vi "Orca Flash Data Spooler.vi"(7 "Calling VI Ref":refnum<vi>) -> ()   [LabVIEW 2016]
uses:
  <vilib>/vision/Image Controls.llb/IMAQ Image.ctl
  Orca Flash Capture Manager Controls/Orca Flash Capture Notifier Type.ctl
  Orca Flash Capture Manager Controls/Orca Flash Capture Actions.ctl
  Orca Flash Capture Manager Controls/Orca Flash Capture Switch Line Scan Modes.ctl
  Orca Flash Data Spooler/Orca Data Spooler Type Defs/Orca Data Spooler Notifier Type.ctl
  Orca Flash Data Spooler/Orca Data Spooler Type Defs/Orca Data Spooler Actions.ctl
  <vilib>/Utility/miscctls.llb/LVPointTypeDef.ctl
  Orca Flash Data Spooler/Orca Data Spooler Type Defs/Orca Data Spooler Last Used.ctl
  Tools/Copy File with Progress/Copy File DLL/x64/Debug/Copy File DLL.dll
panel:
  out "Transfer Amount (%)":u8
  out "Current File":string
  out "Copy Success":bool
  in  "Abort":bool
  in  "Skip File":bool
  in  "Auto Match Paths":bool=TRUE
  in  "Disable Spooler":bool
  in  "Set Destination":bool
  in  "Quit":bool
  out "Destination Path":string
  out "Source Path":string
  out "Start Up Error":errorcluster
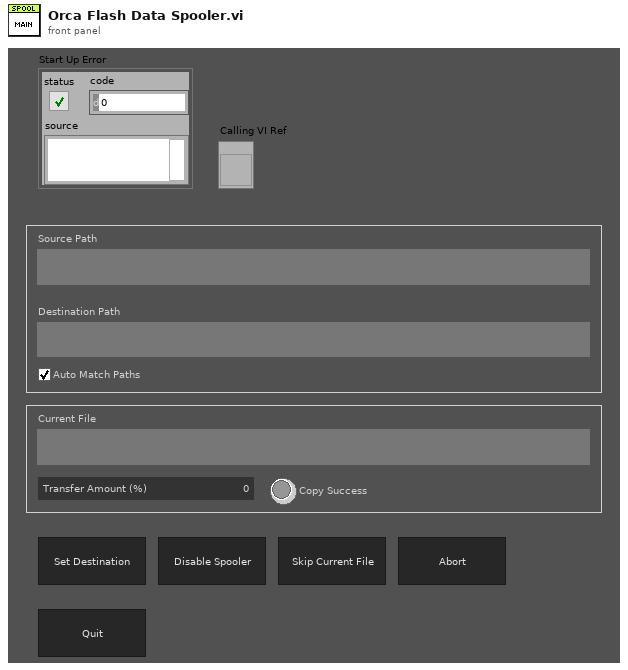
[diagram p1: front panel]
types:
  T1 = enum16{"Always On", "Always Off", "Off While Running"}
  T2 = typedef "LVPointTypeDef.ctl" = cluster{"Horizontal":i16, "Vertical":i16}
  T3 = typedef "Orca Data Spooler Actions.ctl" = enum16{"Idle", "Start Spooler", "Update Destination", "Wait for File", "Copy File", "Copy JSON Files", "Abort", "Exit", "Quit"}
  T4 = typedef "Orca Data Spooler Notifier Type.ctl" = cluster{"Actions":T3, "Source":path, "Destination":path, "Running?":bool}
  T5 = enum8{"Enabled", "Disabled", "Disabled and Grayed Out"}
  T6 = typedef "Orca Flash Capture Notifier Type.ctl" = cluster{"Actions":T7, "Running?":bool, "Preview Exposure (s)":dbl, "Capture Exposure (s)":dbl, "Cycles":u16, "Frames":u32, "No. of Z Steps":u16, "Z Step Size (µm)":dbl, "Base Path":path, "Init Z Position (µm)":dbl, "Lasers Lines":string[], "Save Path":path, "Line Scan?":bool, "Line Scan Mode":T8, "Collect Metadata?":bool}
  T7 = typedef "Orca Flash Capture Actions.ctl" = enum16{"Idle", "Live Preview", "Capture", "Laser On", "Laser Off", "Open Shutters", "Close Shutters", "Set Exposure Time", "Start Acquisition", "Update SubFolder", "Write Metadata", "Setup", "Camera", "Switch", "Step", "Cycle", "External Cycle Sync", "Abort", "Quit"}
  T8 = typedef "Orca Flash Capture Switch Line Scan Modes.ctl" = enum32{"Automatic", "Use Presets", "Manual"}
  T9 = typedef "IMAQ Image.ctl" = refnum<image>
  T10 = cluster{"Image Ref":T9, "Cycle Number":u16, "Camera Running?":bool, "Capture?":bool}
  T11 = enum32{"Bad", "Idle", "Run top level", "Running"}
  T12 = typedef "Orca Data Spooler Last Used.ctl" = cluster{"Source":string, "Destination":string}
  T13 = typedef "LVRectTypeDef.ctl" = cluster{"Left":i16, "Top":i16, "Right":i16, "Bottom":i16}
  T14 = typedef "LVBoundsTypeDef.ctl" = cluster{"Width":u32, "Height":u32}
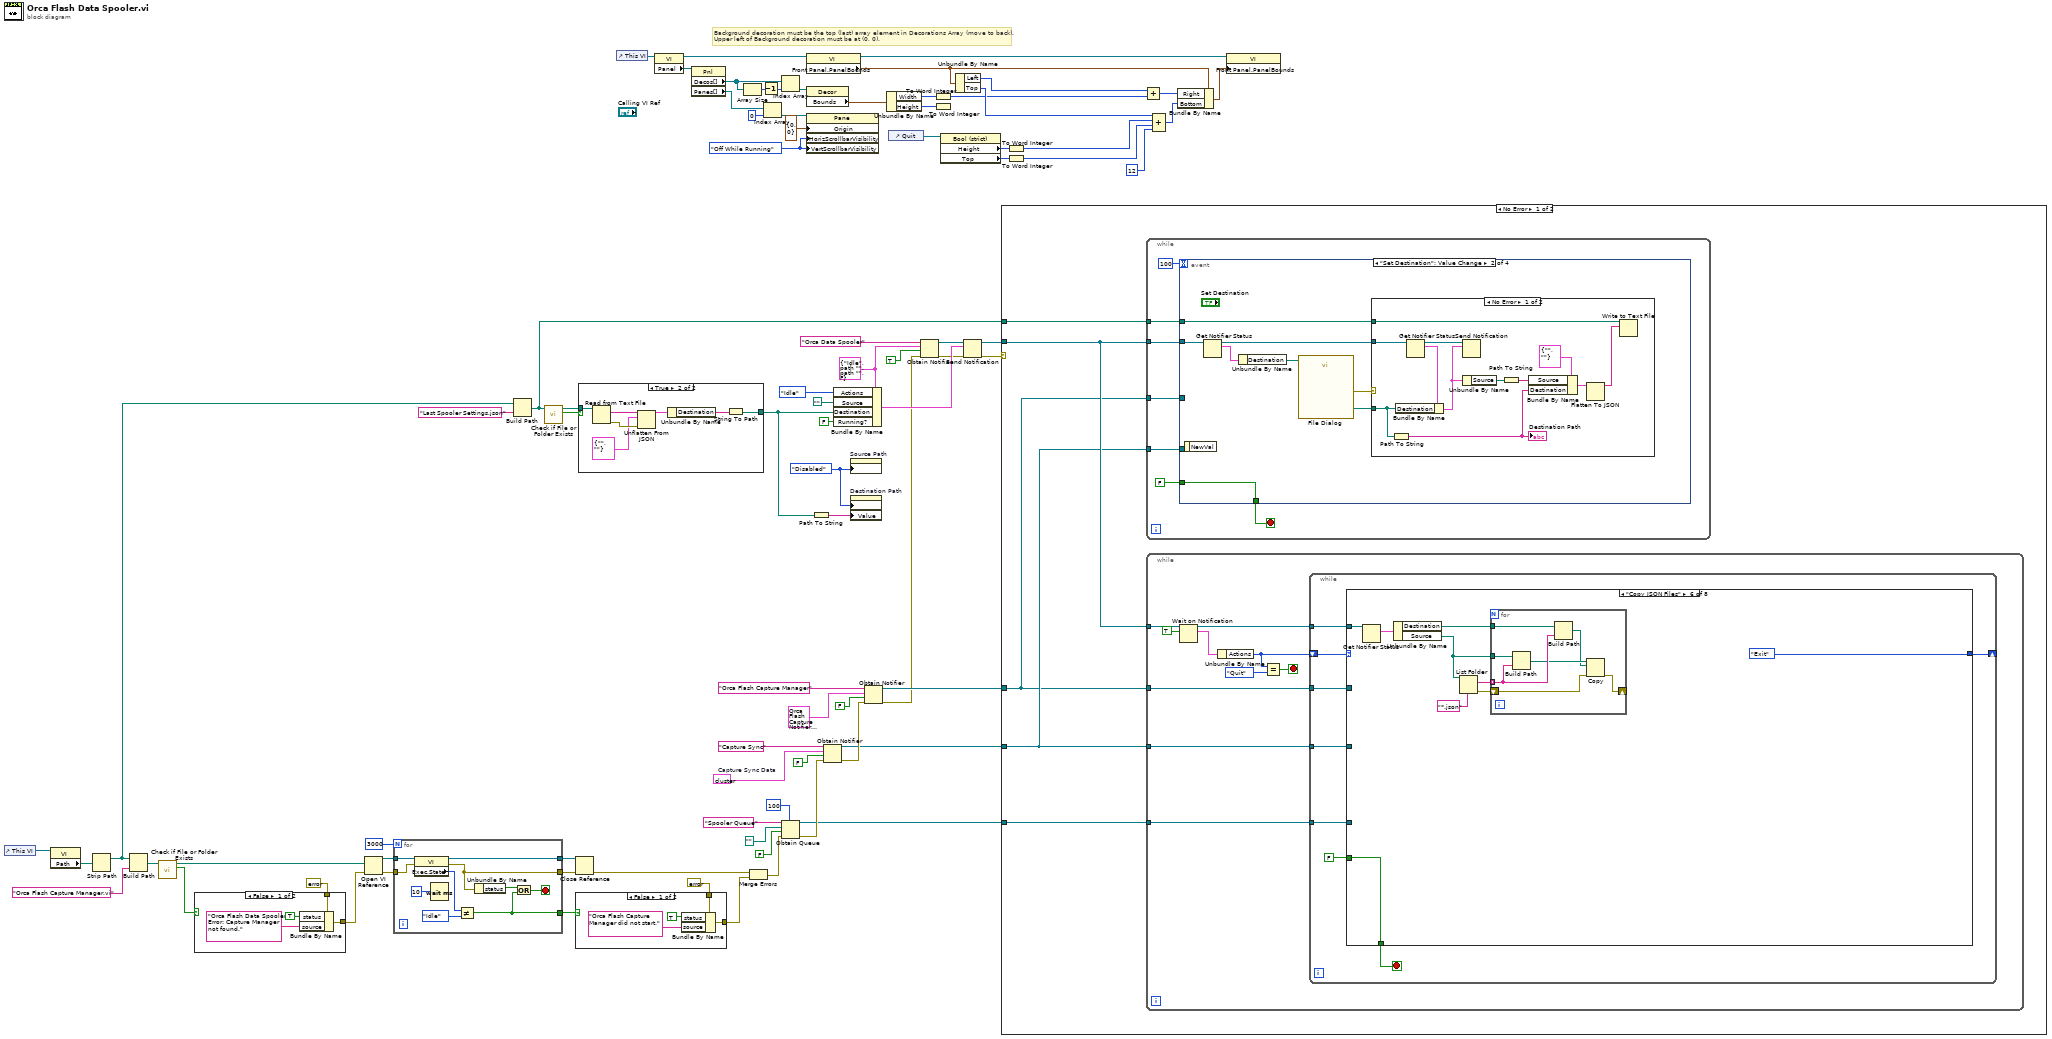
[diagram p0: block diagram]
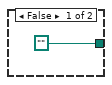
[diagram p2: hidden frame]
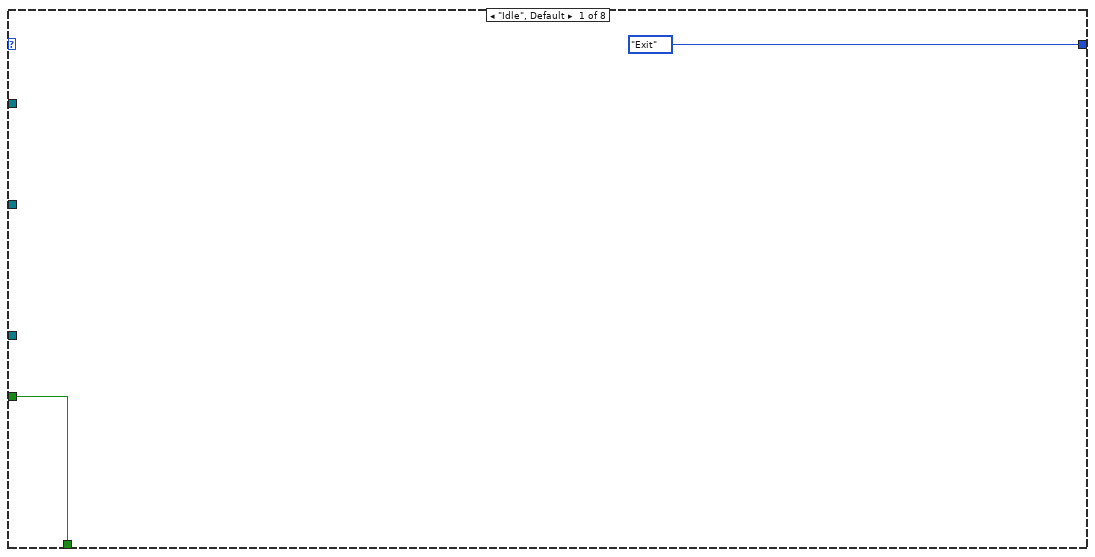
[diagram p3: hidden frame]
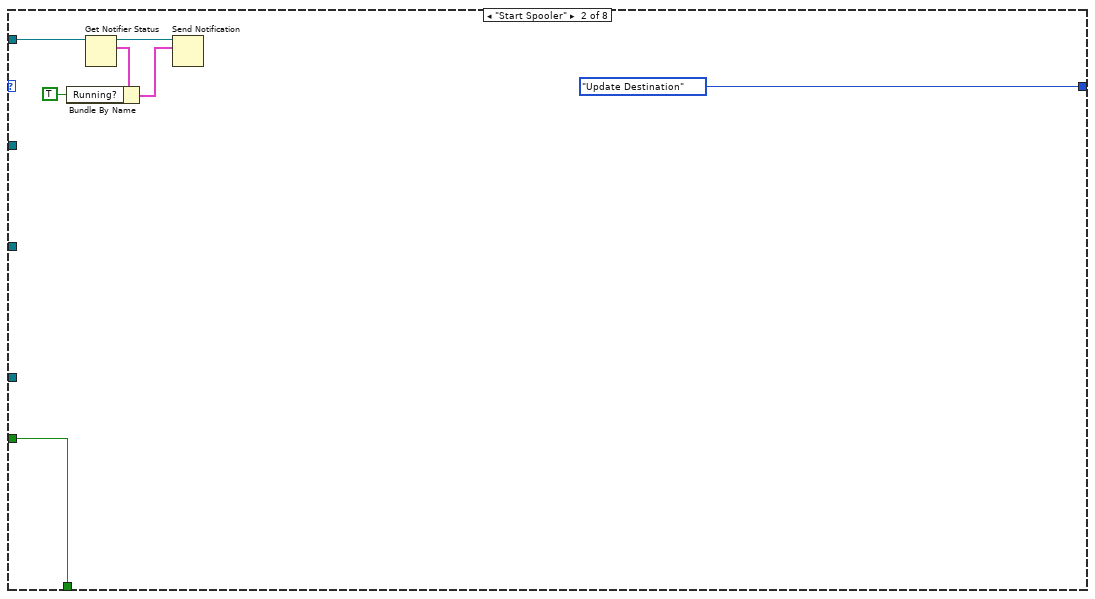
[diagram p4: hidden frame]
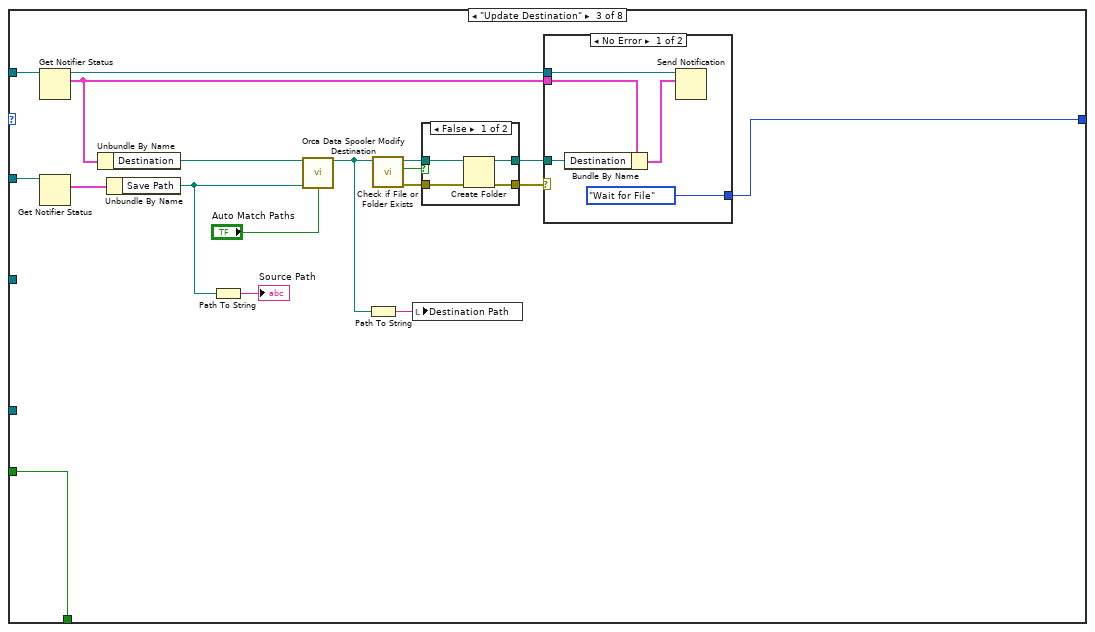
[diagram p5: hidden frame]
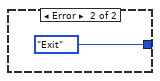
[diagram p6: hidden frame]
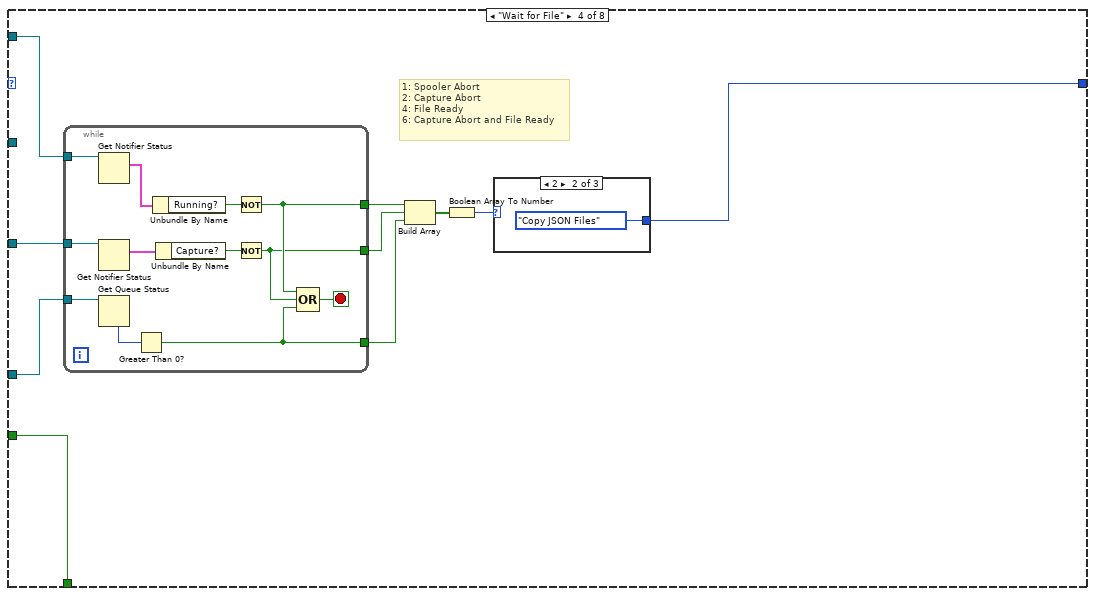
[diagram p8: hidden frame]
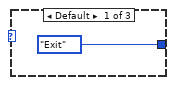
[diagram p9: hidden frame]
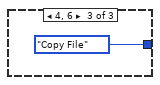
[diagram p10: hidden frame]
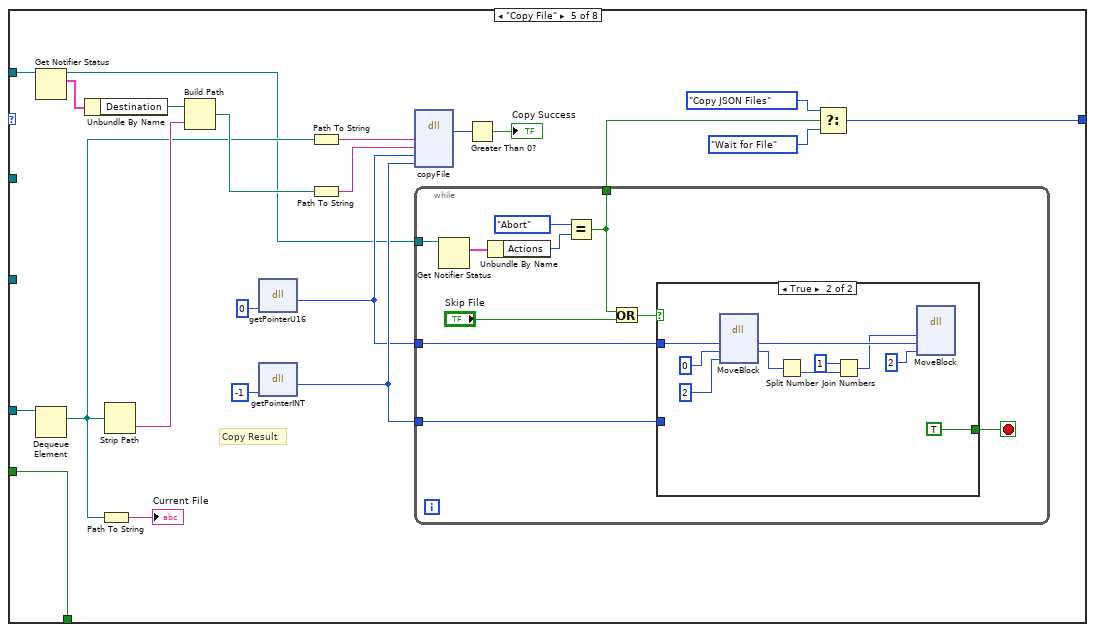
[diagram p11: hidden frame]
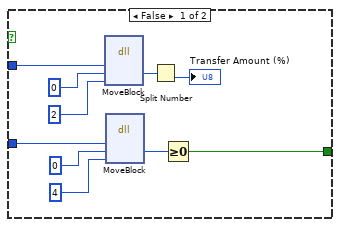
[diagram p12: hidden frame]
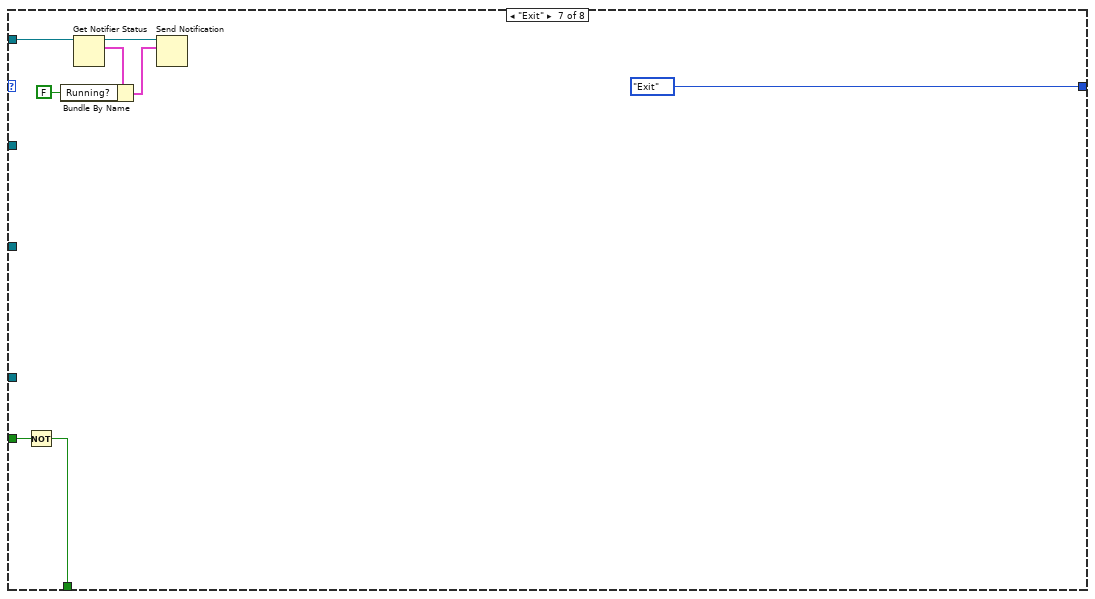
[diagram p13: hidden frame]
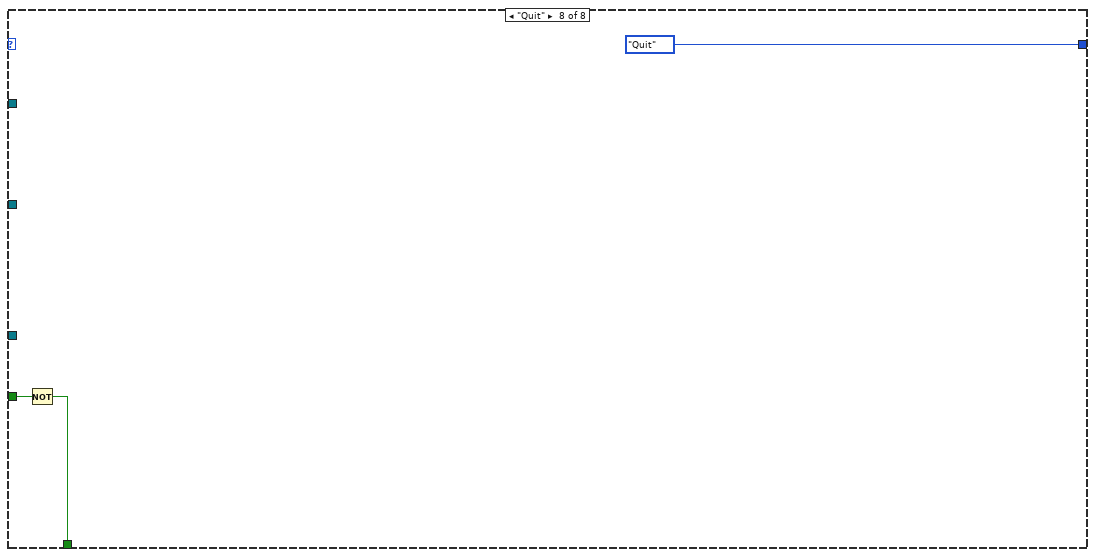
[diagram p14: hidden frame]
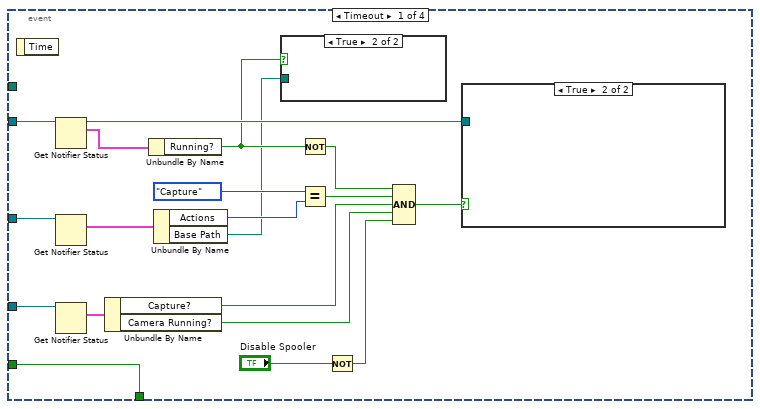
[diagram p15: hidden frame]
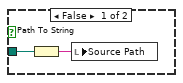
[diagram p16: hidden frame]
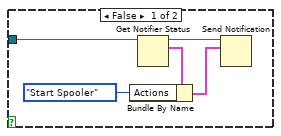
[diagram p17: hidden frame]
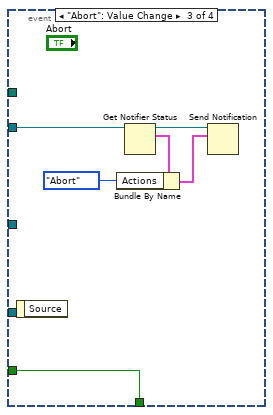
[diagram p19: hidden frame]
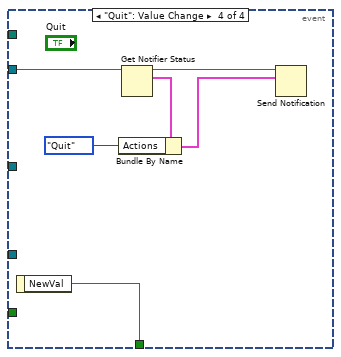
[diagram p20: hidden frame]
diagram:
  w21 = T1."Off While Running" ("Vertical Scrollbar Visibility")
  w47 = T4 {"Actions"=enum."Idle", "Source"=path "", "Destination"=path "", "Running?"=FALSE} ("Orca Data Spooler Notifier Type")
  w54 = T5."Disabled" ("Disabled")
  w69 = T10 {"Image Ref"=refnum, "Cycle Number"=0, "Camera Running?"=FALSE, "Capture?"=FALSE}  # Capture Sync Data
  # "Background decoration must be the top (last) array element in Decorations Array (move to back).\nUpper left of Background decoration must be at (0, 0)."
  n1 = control-ref of="This VI"() -> (w82:refnum<vi>)
  n2 = property class="VI"(reference=w82) -> ("Path"=w81:path)  [unwired: 1 in, 2 out]
  n3 = Strip Path(path=w81) -> (stripped path=w52:path)  [unwired: 1 out]
  n4 = Build Path(base path=w52, name or relative path="Orca Flash Capture Manager.vi" ("name (unnamed)")) -> (appended path=w79:path)
  n5 = call <vilib>:"Check if File or Folder Exists.vi"("path"=w79) -> ("file or folder exists?"=w78:bool, "dup path"=w75:path)  [unwired: 8 in, 1 out]
  n6 = case shown="False" w78 {
    tunnel: errorcluster {"status"=FALSE, "code"=0, "source"=""} ("error in (no error)") -> [w84 w87]
    tunnel: [w83 w87] -> w74
    frame False {
      n7 = Bundle By Name(cluster=w84, "status"=TRUE, "source"="Orca Flash Data Spooler Error: Capture Manager not found." ("name (unnamed)")) -> (w83:errorcluster)
    }
    frame True {
    }
  }
  n8 = Open VI Reference(vi path=w75, error in (no error)=w74) -> (vi reference=w76:refnum<vi>, error out=w70:errorcluster)  [unwired: 4 in]
  n9 = for {
    N: 3000 -> [_]
    tunnel: w76 -> [w97]
    tunnel: [w93] -> w72
    tunnel: [w88] -> w62
    tunnel: [w90] -> w71
    tunnel: w70 -> [w89]
    stop <- w91 stop-if-true
    n10 = property class="VI"(reference=w97, error in=w89) -> (reference out=w93:refnum<vi>, error out=w90:errorcluster, "Exec.State"=w95:T11)
    n11 = Wait (ms)(milliseconds to wait=u32 10) -> ()  [unwired: 1 out]
    n12 = Not Equal?(x=w95, y=T11."Idle") -> (x != y?=w88:bool)
    n13 = Unbundle By Name(w90) -> ("status"=w92:bool)
    n14 = Or(x=w92, y=w88) -> (x .or. y?=w91:bool)
  }
  n15 = Build Path(base path=w52, name or relative path="Last Spooler Settings.json" ("name (unnamed)")) -> (appended path=w1:path)
  n16 = call <vilib>:"Check if File or Folder Exists.vi"("path"=w1) -> ("file or folder exists?"=w50:bool, "dup path"=w51:path)  [unwired: 8 in, 1 out]
  n17 = Close Reference(reference=w72, error in (no error)=w71) -> (error out=w61:errorcluster)
  n18 = case shown="False" w62 {
    tunnel: errorcluster {"status"=FALSE, "code"=0, "source"=""} ("error in (no error)") -> [w99 w102]
    tunnel: [w98 w102] -> w60
    frame False {
      n19 = Bundle By Name(cluster=w99, "status"=TRUE, "source"="Orca Flash Capture Manager did not start." ("name (unnamed)")) -> (w98:errorcluster)
    }
    frame True {
    }
  }
  n20 = case shown="True" w50 {
    tunnel: w51 -> [_ w108]
    tunnel: [path "" w104] -> w43
    frame False {
    }
    frame True {
      n21 = Read from Text File(file (use dialog)=w108) -> (text=w110:string, error out=w109:errorcluster)  [unwired: 3 in, 2 out]
      n22 = Unflatten From JSON(JSON string=w110, type and defaults=T12 {"Source"="", "Destination"=""} ("Orca Data Spooler Notifier Type"), error in (no error)=w109) -> (value=w106:T12)  [unwired: 4 in, 1 out]
      n23 = Unbundle By Name(w106) -> ("Destination"=w105:string)
      n24 = String To Path(string=w105) -> (path=w104:path)
    }
  }
  n25 = control-ref of="This VI"() -> (w13:refnum<vi>)
  n26 = property class="VI"(reference=w13) -> (reference out=w22:refnum<vi>, "Panel"=w14:refnum<vi>)  [unwired: 1 in, 1 out]
  n27 = property class="Pnl"(reference=w14) -> ("Decos[]"=w12:refnum<vi>[], "Panes[]"=w18:refnum<vi>[])  [unwired: 1 in, 2 out]
  n28 = Array Size(array=w12) -> (size(s)=w10:i32)
  n29 = Merge Errors(w61, w60) -> (w4:errorcluster)
  n30 = Decrement(x=w10) -> (x-1=w11:i32)
  n31 = Index Array(array=w18, index=0) -> (element=w17:refnum<vi>)
  n32 = Index Array(array=w12, index=w11) -> (element=w20:refnum<vi>)
  n33 = Obtain Queue(max queue size (-1, unlimited)=100, name (unnamed)="Spooler Queue", element data type=path "", create if not found? (T)=FALSE, error in (no error)=w4) -> (queue out=w2:refnum<queue>, error out=w3:errorcluster)  [unwired: 1 out]
  n34 = property class="VI"(reference=w22) -> (reference out=w24:refnum<vi>, "Front Panel.PanelBounds"=w25:T13)  [unwired: 1 in, 1 out]
  n35 = property class="Decor"(reference=w20) -> ("Bounds"=w23:T14)  [unwired: 1 in, 2 out]
  n36 = property class="Pane"(reference=w17, "Origin"=T2 {"Horizontal"=0, "Vertical"=0}, "HorizScrollbarVisibility"=w21, "VertScrollbarVisibility"=w21) -> ()  [unwired: 1 in, 2 out]
  n37 = Path To String(path=w43) -> (string=w42:string)
  n38 = Obtain Notifier(name (unnamed)="Capture Sync", notification data type=w69, create if not found? (T)=FALSE, error in (no error)=w3) -> (notifier out=w57:refnum<notifier>, error out=w59:errorcluster)  [unwired: 1 out]
  n39 = Bundle By Name(cluster=w47, "Actions"=Orca_Data_Spooler_Actions."Idle", "Source"=path "", "Destination"=w43, "Running?"=FALSE) -> (w45:T4)
  n40 = property on="Source Path" class="Str"("DisabledEnum"=w54) -> ()  [unwired: 2 in, 2 out]
  n41 = property on="Destination Path" class="Str"("DisabledEnum"=w54, "Value"=w42) -> ()  [unwired: 2 in, 2 out]
  n42 = Obtain Notifier(name (unnamed)="Orca Flash Capture Manager", notification data type=T6 {"Actions"=enum."Live Preview", "Running?"=FALSE, "Preview Exposure (s)"=0.1, "Capture Exposure (s)"=0.1, "Cycles"=1, "Frames"=0, "No. of Z Steps"=0, "Z Step Size (µm)"=0.0, "Base Path"=path "", "Init Z Position (µm)"=0.0, "Lasers Lines"=[], "Save Path"=path "", "Line Scan?"=FALSE, "Line Scan Mode"=enum."Automatic", "Collect Metadata?"=FALSE} ("4Pi Capture Notifier Type"), create if not found? (T)=FALSE, error in (no error)=w59) -> (notifier out=w58:refnum<notifier>, error out=w41:errorcluster)  [unwired: 1 out]
  n43 = Unbundle By Name(w23) -> ("Width"=w28:u32, "Height"=w31:u32)
  n44 = control-ref of="Quit"() -> (w15:refnum<vi>)
  n45 = Obtain Notifier(name (unnamed)="Orca Data Spooler", notification data type=w47, create if not found? (T)=TRUE, error in (no error)=w41) -> (notifier out=w46:refnum<notifier>, error out=w44:errorcluster)  [unwired: 1 out]
  n46 = To Word Integer(number=w28) -> (16bit integer=w30:i16)
  n47 = To Word Integer(number=w31) -> ()  [unwired: 1 out]
  n48 = property class="Bool (strict)"(reference=w15) -> ("Height"=w33:u32, "Top"=w34:i32)  [unwired: 1 in, 2 out]
  n49 = Unbundle By Name(w25) -> ("Left"=w27:i16, "Top"=w38:i16)
  n50 = Send Notification(notification=w45, notifier=w46, error in (no error)=w44) -> (notifier out=w39:refnum<notifier>, error out=w40:errorcluster)
  n51 = case shown="No Error" w40 {
    selector: w40 -> [_ w348]
    tunnel: w58 -> [w113 w346]
    tunnel: w57 -> [w114 w344]
    tunnel: w39 -> [w115 w345]
    tunnel: w2 -> [w112 _]
    tunnel: w1 -> [w111 _]
    frame No Error {
      n52 = while {
        tunnel: w115 -> [w281]
        tunnel: w113 -> [w280]
        tunnel: w114 -> [w279]
        tunnel: w111 -> [w277]
        stop <- w282 stop-if-true
        n53 = event shown="[1] \"Set Destination\": Value Change" {
          selector: _ -> [_ _ _ _]
          dyn-events: _ -> [_ _ _ _]
          timeout: 100 -> [_ _ _ _]
          tunnel: FALSE -> [w302 w317 w335 _]
          tunnel: [w302 w317 w335 w341] -> w282
          tunnel: w281 -> [w291 w316 w331 w340]
          tunnel: w280 -> [w301 _ _ _]
          tunnel: w279 -> [w300 _ _ _]
          tunnel: w277 -> [_ w310 _ _]
          event Timeout {
            n54 = event-data() -> ()  [unwired: 1 in, 1 out]
            n55 = Get Notifier Status(notifier=w291) -> (notifier out=w288:refnum<notifier>, current notification=w290:T4)  [unwired: 1 in, 3 out]
            n56 = Get Notifier Status(notifier=w301) -> (current notification=w299:T6)  [unwired: 1 in, 4 out]
            n57 = Get Notifier Status(notifier=w300) -> (current notification=w296:T10)  [unwired: 1 in, 4 out]
            n58 = Unbundle By Name(w296) -> ("Capture?"=w293:bool, "Camera Running?"=w294:bool)
            n59 = Unbundle By Name(w290) -> ("Running?"=w285:bool)
            n60 = Unbundle By Name(w299) -> ("Actions"=w298:T7, "Base Path"=w284:path)
            n61 = case shown="True" w285 {
              tunnel: w284 -> [w303 _]
              frame False {
                n62 = Path To String(path=w303) -> (string=w304:string)
                n63 = local write "Source Path"(w304) -> ()
              }
              frame True {
              }
            }
            n64 = Not(x=w285) -> (.not. x?=w289:bool)
            n65 = Equal?(x=Orca_Flash_Capture_Actions."Capture", y=w298) -> (x = y?=w295:bool)
            n66 = Not(x="Disable Spooler") -> (.not. x?=w286:bool)
            n67 = Compound Arithmetic op=AND(w289, w295, w293, w294, w286) -> (w292:bool)
            n68 = case shown="True" w292 {
              tunnel: w288 -> [w309 _]
              frame False {
                n69 = Get Notifier Status(notifier=w309) -> (notifier out=w308:refnum<notifier>, current notification=w307:T4)  [unwired: 1 in, 3 out]
                n70 = Bundle By Name(cluster=w307, "Actions"=Orca_Data_Spooler_Actions."Start Spooler") -> (w306:T4)
                n71 = Send Notification(notification=w306, notifier=w308) -> ()  [unwired: 1 in, 2 out]
              }
              frame True {
              }
            }
          }
          event "Set Destination": Value Change {
            n72 = event-data() -> ()  [unwired: 1 in, 1 out]
            n73 = Get Notifier Status(notifier=w316) -> (notifier out=w312:refnum<notifier>, current notification=w315:T4)  [unwired: 1 in, 3 out]
            n74 = Unbundle By Name(w315) -> ("Destination"=w314:path)
            n75 = call "File Dialog"("start path"=w314) -> ("selected path"=w311:path, "error out"=w313:errorcluster)  [unwired: 11 in, 2 out]
            n76 = case shown="No Error" w313 {
              tunnel: w312 -> [w329 _]
              tunnel: w311 -> [w327 _]
              tunnel: w310 -> [w325 _]
              frame No Error {
                n77 = Path To String(path=w327) -> (string=w322:string)
                "Destination Path" <- w322
                n78 = Get Notifier Status(notifier=w329) -> (notifier out=w326:refnum<notifier>, current notification=w328:T4)  [unwired: 1 in, 3 out]
                n79 = Bundle By Name(cluster=w328, "Destination"=w327) -> (w321:T4)
                n80 = Send Notification(notification=w321, notifier=w326) -> ()  [unwired: 1 in, 2 out]
                n81 = Unbundle By Name(w321) -> ("Source"=w319:path)
                n82 = Path To String(path=w319) -> (string=w320:string)
                n83 = Bundle By Name(cluster=T12 {"Source"="", "Destination"=""} ("Orca Data Spooler Notifier Type"), "Source"=w320, "Destination"=w322) -> (w324:T12)
                n84 = Flatten To JSON(anything=w324) -> (JSON string=w318:string)  [unwired: 2 in, 1 out]
                n85 = Write to Text File(file (use dialog)=w325, text=w318) -> ()  [unwired: 2 in, 3 out]
              }
              frame Error {
              }
            }
          }
          event "Abort": Value Change {
            n86 = event-data() -> ()  [unwired: 1 in, 1 out]
            n87 = Get Notifier Status(notifier=w331) -> (notifier out=w334:refnum<notifier>, current notification=w333:T4)  [unwired: 1 in, 3 out]
            n88 = Bundle By Name(cluster=w333, "Actions"=Orca_Data_Spooler_Actions."Abort") -> (w332:T4)
            n89 = Send Notification(notification=w332, notifier=w334) -> ()  [unwired: 1 in, 2 out]
          }
          event "Quit": Value Change {
            n90 = event-data() -> ("NewVal"=w341:bool)  [unwired: 1 in]
            n91 = Get Notifier Status(notifier=w340) -> (notifier out=w338:refnum<notifier>, current notification=w339:T4)  [unwired: 1 in, 3 out]
            n92 = Bundle By Name(cluster=w339, "Actions"=Orca_Data_Spooler_Actions."Quit") -> (w337:T4)
            n93 = Send Notification(notification=w337, notifier=w338) -> ()  [unwired: 1 in, 2 out]
          }
        }
      }
      n94 = while {
        tunnel: w115 -> [w125]
        tunnel: w114 -> [w118]
        tunnel: w113 -> [w117]
        tunnel: w112 -> [w116]
        stop <- w121 stop-if-true
        n95 = Wait on Notification(notifier=w125, ignore previous (F)=TRUE) -> (notifier out=w119:refnum<notifier>, notification=w123:T4)  [unwired: 2 in, 2 out]
        n96 = Unbundle By Name(w123) -> ("Actions"=w120:T3)
        n97 = Equal?(x=w120, y=Orca_Data_Spooler_Actions."Quit") -> (x = y?=w121:bool)
        n98 = while {
          shift-right: [w129] -> _
          shift-left: w120 -> [w133]
          tunnel: w119 -> [w132]
          tunnel: w118 -> [w128]
          tunnel: w117 -> [w127]
          tunnel: w116 -> [w126]
          stop <- w130 stop-if-true
          n99 = case shown="\"Copy JSON Files\"" w133 {
            tunnel: w132 -> [_ w140 w157 w180 w209 w257 w267 _]
            tunnel: FALSE -> [w135 w142 w160 w182 w219 w258 w273 w276]
            tunnel: [w135 w142 w160 w182 w219 w258 w272 w275] -> w130
            tunnel: [Orca_Data_Spooler_Actions."Exit" ("y") Orca_Data_Spooler_Actions."Update Destination" ("y") w143 w173 w199 Orca_Data_Spooler_Actions."Exit" ("y") Orca_Data_Spooler_Actions."Exit" ("y") Orca_Data_Spooler_Actions."Quit" ("y")] -> w129
            tunnel: w128 -> [_ _ _ w179 _ _ _ _]
            tunnel: w127 -> [_ _ w159 _ _ _ _ _]
            tunnel: w126 -> [_ _ _ w181 w210 _ _ _]
            frame "Idle", Default {
            }
            frame "Start Spooler" {
              n100 = Get Notifier Status(notifier=w140) -> (notifier out=w138:refnum<notifier>, current notification=w139:T4)  [unwired: 1 in, 3 out]
              n101 = Bundle By Name(cluster=w139, "Running?"=TRUE) -> (w136:T4)
              n102 = Send Notification(notification=w136, notifier=w138) -> ()  [unwired: 1 in, 2 out]
            }
            frame "Update Destination" {
              n103 = Get Notifier Status(notifier=w157) -> (notifier out=w155:refnum<notifier>, current notification=w154:T4)  [unwired: 1 in, 3 out]
              n104 = Get Notifier Status(notifier=w159) -> (current notification=w158:T6)  [unwired: 1 in, 4 out]
              n105 = Unbundle By Name(w154) -> ("Destination"=w152:path)
              n106 = Unbundle By Name(w158) -> ("Save Path"=w151:path)
              n107 = Path To String(path=w151) -> (string=→"Source Path":string)
              n108 = call "Orca Data Spooler Modify Destination.vi"("Destination"=w152, "Source"=w151, "Ignore Source?"="Auto Match Paths") -> ("Modified Destination"=w149:path)  [unwired: 12 in]
              n109 = Path To String(path=w149) -> (string=w153:string)
              n110 = call <vilib>:"Check if File or Folder Exists.vi"("path"=w149) -> ("error out"=w146:errorcluster, "file or folder exists?"=w148:bool, "dup path"=w147:path)  [unwired: 8 in]
              n111 = local write "Destination Path"(w153) -> ()
              n112 = case shown="False" w148 {
                tunnel: w147 -> [w170 w171]
                tunnel: w146 -> [w169 w172]
                tunnel: [w168 w172] -> w145
                tunnel: [w167 w171] -> w144
                frame False {
                  n113 = Create Folder(path (use dialog)=w170, error in=w169) -> (created path=w167:path, error out=w168:errorcluster)  [unwired: 1 in, 1 out]
                }
                frame True {
                }
              }
              n114 = case shown="No Error" w145 {
                tunnel: w155 -> [w165 _]
                tunnel: w154 -> [w164 _]
                tunnel: w144 -> [w162 _]
                tunnel: [Orca_Data_Spooler_Actions."Wait for File" ("y") Orca_Data_Spooler_Actions."Exit" ("y")] -> w143
                frame No Error {
                  n115 = Bundle By Name(cluster=w164, "Destination"=w162) -> (w163:T4)
                  n116 = Send Notification(notification=w163, notifier=w165) -> ()  [unwired: 1 in, 2 out]
                }
                frame Error {
                }
              }
            }
            frame "Wait for File" {
              # "1: Spooler Abort\n2: Capture Abort\n4: File Ready\n6: Capture Abort and File Ready"
              n117 = while {
                tunnel: w181 -> [w196]
                tunnel: w180 -> [w197]
                tunnel: [w187] -> w178
                tunnel: w179 -> [w193]
                tunnel: [w186] -> w176
                tunnel: [w190] -> w177
                stop <- w191 stop-if-true
                n118 = Get Notifier Status(notifier=w197) -> (current notification=w194:T4)  [unwired: 1 in, 4 out]
                n119 = Get Notifier Status(notifier=w193) -> (current notification=w192:T10)  [unwired: 1 in, 4 out]
                n120 = Get Queue Status(queue=w196) -> (# elements in queue=w195:i32)  [unwired: 2 in, 7 out]
                n121 = Greater Than 0?(x=w195) -> (x > 0?=w190:bool)
                n122 = Unbundle By Name(w194) -> ("Running?"=w188:bool)
                n123 = Unbundle By Name(w192) -> ("Capture?"=w189:bool)
                n124 = Not(x=w188) -> (.not. x?=w187:bool)
                n125 = Not(x=w189) -> (.not. x?=w186:bool)
                n126 = Compound Arithmetic op=OR(w187, w186, w190) -> (w191:bool)
              }
              n127 = Build Array(w178, w176, w177) -> (w175:bool[])
              n128 = Boolean Array To Number(Boolean array=w175) -> (number=w174:u32)
              n129 = case shown="2" w174 {
                tunnel: [Orca_Data_Spooler_Actions."Exit" ("y") Orca_Data_Spooler_Actions."Copy JSON Files" ("y") Orca_Data_Spooler_Actions."Copy File" ("y")] -> w173
                frame Default {
                }
                frame 2 {
                }
                frame 4, 6 {
                }
              }
            }
            frame "Copy File" {
              # "Copy Result"
              n130 = Get Notifier Status(notifier=w209) -> (notifier out=w202:refnum<notifier>, current notification=w208:T4)  [unwired: 1 in, 3 out]
              n131 = Dequeue Element(queue=w210) -> (element=w204:path)  [unwired: 2 in, 3 out]
              n132 = Unbundle By Name(w208) -> ("Destination"=w207:path)
              n133 = Path To String(path=w204) -> (string=→"Current File":string)
              n134 = Strip Path(path=w204) -> (name=w206:string)  [unwired: 1 out]
              n135 = Build Path(base path=w207, name or relative path=w206) -> (appended path=w205:path)
              n136 = dll-call lib="D:/Microscope-Control/Tools/Copy File with Progress/Copy File DLL/x64/Debug/Copy File DLL.dll" fn="getPointerU16"("Variable"=u16 0) -> ("Pointer Value"=w216:u64)  [unwired: 4 in, 2 out]
              n137 = dll-call lib="D:/Microscope-Control/Tools/Copy File with Progress/Copy File DLL/x64/Debug/Copy File DLL.dll" fn="getPointerINT"("Variable"=-1) -> ("Pointer Value"=w218:u64)  [unwired: 4 in, 2 out]
              n138 = Path To String(path=w204) -> (string=w215:string)
              n139 = Path To String(path=w205) -> (string=w214:string)
              n140 = dll-call lib="D:/Microscope-Control/Tools/Copy File with Progress/Copy File DLL/x64/Debug/Copy File DLL.dll" fn="copyFile"("Source File"=w215, "Destination File"=w214, "Update Value Pointer"=w216, "Copy Result Pointer"=w218) -> ("Success"=w213:i32)  [unwired: 7 in, 2 out]
              n141 = while {
                tunnel: w216 -> [w229]
                tunnel: w218 -> [w228]
                tunnel: w202 -> [w226]
                tunnel: [w221] -> w201
                stop <- w227 stop-if-true
                n142 = Get Notifier Status(notifier=w226) -> (current notification=w225:T4)  [unwired: 1 in, 4 out]
                n143 = Unbundle By Name(w225) -> ("Actions"=w224:T3)
                n144 = Equal?(x=Orca_Data_Spooler_Actions."Abort", y=w224) -> (x = y?=w221:bool)
                n145 = Or(x=w221, y="Skip File") -> (x .or. y?=w222:bool)
                n146 = case shown="True" w222 {
                  tunnel: w229 -> [w239 w241]
                  tunnel: w228 -> [w238 _]
                  tunnel: [w237 TRUE] -> w227
                  frame False {
                    n147 = dll-call lib="LabVIEW" fn="MoveBlock"("Pointer to Source"=w239, "Destination"=u16 0, "Bytes to Move"=2) -> ("Destination"=w234:u16)  [unwired: 6 in, 2 out]
                    n148 = dll-call lib="LabVIEW" fn="MoveBlock"("Pointer to Source"=w238, "Destination"=0, "Bytes to Move"=4) -> ("Destination"=w231:i32)  [unwired: 6 in, 2 out]
                    n149 = Split Number(x=w234) -> (lo(x)=→"Transfer Amount (%)":u8)  [unwired: 1 out]
                    n150 = Greater Or Equal To 0?(x=w231) -> (x >= 0?=w237:bool)
                  }
                  frame True {
                    n151 = dll-call lib="LabVIEW" fn="MoveBlock"("Pointer to Source"=w241, "Destination"=u16 0, "Bytes to Move"=2) -> ("Pointer to Source"=w243:u64, "Destination"=w247:u16)  [unwired: 5 in, 2 out]
                    n152 = Split Number(x=w247) -> (lo(x)=w246:u8)  [unwired: 1 out]
                    n153 = Join Numbers(hi=u8 1, lo=w246) -> ((hi.lo)=w242:u16)
                    n154 = dll-call lib="LabVIEW" fn="MoveBlock"("Source"=w242, "Destination Pointer"=w243, "Bytes to Move"=2) -> ()  [unwired: 7 in, 2 out]
                  }
                }
              }
              n155 = Greater Than 0?(x=w213) -> (x > 0?=→"Copy Success":bool)
              n156 = Select(t=Orca_Data_Spooler_Actions."Copy JSON Files", s=w201, f=Orca_Data_Spooler_Actions."Wait for File" ("y")) -> (s? t:f=w199:T3)
            }
            frame "Copy JSON Files" {
              n157 = Get Notifier Status(notifier=w257) -> (current notification=w256:T4)  [unwired: 1 in, 4 out]
              n158 = Unbundle By Name(w256) -> ("Destination"=w252:path, "Source"=w253:path)
              n159 = List Folder(path=w253, pattern="*.json") -> (filenames=w254:string[], error out=w251:errorcluster)  [unwired: 2 in, 2 out]
              n160 = for {
                tunnel: w254 -> [w263] mode=indexing
                tunnel: w253 -> [w265]
                tunnel: w252 -> [w264]
                shift-right: [w259] -> _
                shift-left: w251 -> [w260]
                n161 = Build Path(base path=w265, name or relative path=w263) -> (appended path=w262:path)
                n162 = Build Path(base path=w264, name or relative path=w263) -> (appended path=w261:path)
                n163 = Copy(8:w260, 10:w261, 11:w262) -> (0:w259:errorcluster)  [unwired: 2 in, 2 out]
              }
            }
            frame "Exit" {
              n164 = Not(x=w273) -> (.not. x?=w272:bool)
              n165 = Get Notifier Status(notifier=w267) -> (notifier out=w270:refnum<notifier>, current notification=w269:T4)  [unwired: 1 in, 3 out]
              n166 = Bundle By Name(cluster=w269, "Running?"=FALSE) -> (w268:T4)
              n167 = Send Notification(notification=w268, notifier=w270) -> ()  [unwired: 1 in, 2 out]
            }
            frame "Quit" {
              n168 = Not(x=w276) -> (.not. x?=w275:bool)
            }
          }
        }
      }
    }
    frame Error {
      n169 = Release Notifier(notifier=w345, error in (no error)=w348) -> (error out=w347:errorcluster)  [unwired: 1 in, 2 out]
      n170 = Release Notifier(notifier=w346, error in (no error)=w347) -> (error out=w343:errorcluster)  [unwired: 1 in, 2 out]
      n171 = Release Notifier(notifier=w344, error in (no error)=w343) -> (error out=→"Start Up Error":errorcluster)  [unwired: 1 in, 2 out]
    }
  }
  n172 = To Word Integer(number=w33) -> (16bit integer=w36:i16)
  n173 = To Word Integer(number=w34) -> (16bit integer=w37:i16)
  n174 = Add(x=w27, y=w30) -> (x+y=w29:i16)
  n175 = Compound Arithmetic op=ADD(w38, w36, w37, i16 12 ("y")) -> (w32:i16)
  n176 = Bundle By Name(cluster=w25, "Right"=w29, "Bottom"=w32) -> (w26:T13)
  n177 = property class="VI"(reference=w24, "Front Panel.PanelBounds"=w26) -> ()  [unwired: 1 in, 2 out]
